vi "DB - Sort Item Names To DB.vi"(10 "DB Query Array":string[][](array[string]), 11 "ItemNames":string[][](array[string])) -> (2 "ItemNames":string[][](array[string]), 3 "DB Query Array":string[][](array[string]))   [LabVIEW 2020]
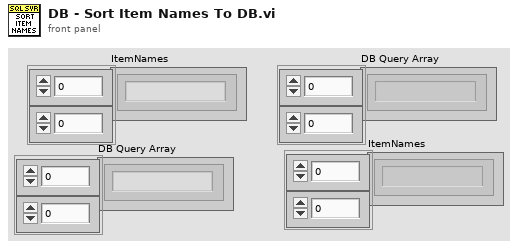
[diagram p1: front panel]
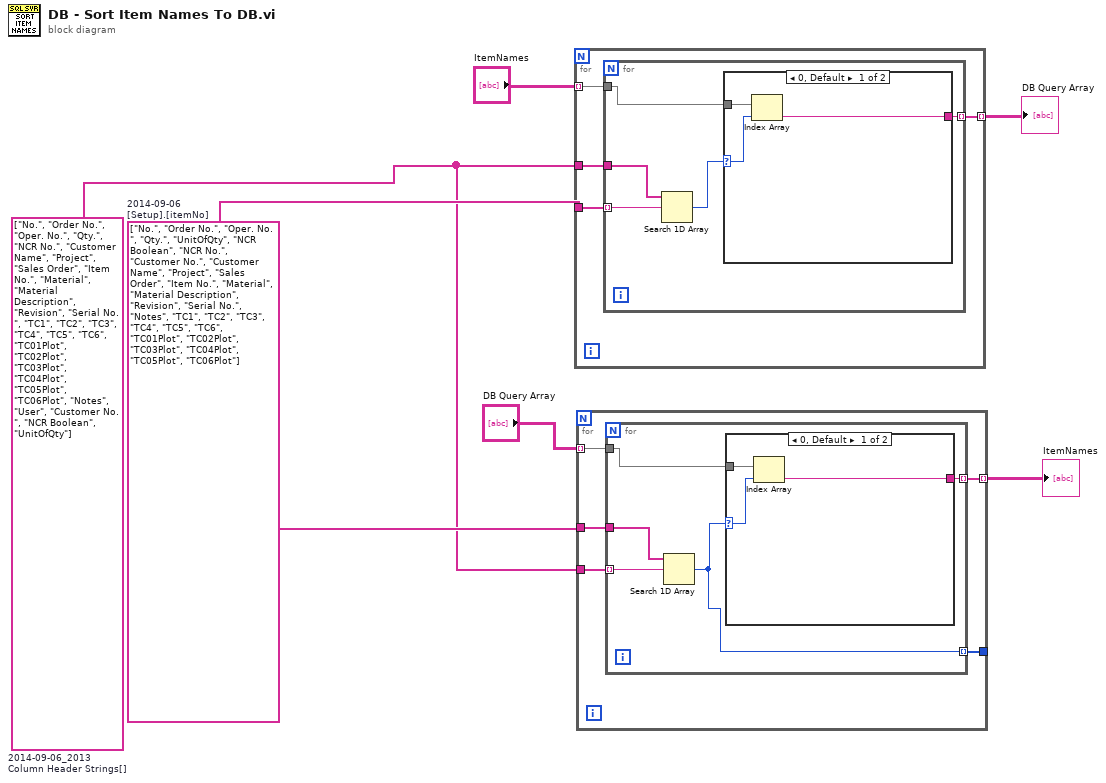
[diagram p0: block diagram]
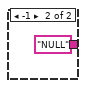
[diagram p2: hidden frame]
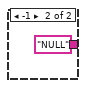
[diagram p3: hidden frame]
diagram:
  w2 = string[] ["No.", "Order No.", "Oper. No.", "Qty.", "NCR No.", "Customer Name", "Project", "Sales Order", "Item No.", "Material", "Material Description", "Revision", "Serial No.", "TC1", "TC2", "TC3", "TC4", "TC5", "TC6", "TC01Plot", "TC02Plot", "TC03Plot", "TC04Plot", "TC05Plot", "TC06Plot", "Notes", "User", "Customer No.", "NCR Boolean", "UnitOfQty"]  # 2014-09-06_2013 Column Header Strings[]
  w3 = string[] ["No.", "Order No.", "Oper. No.", "Qty.", "UnitOfQty", "NCR Boolean", "NCR No.", "Customer No.", "Customer Name", "Project", "Sales Order", "Item No.", "Material", "Material Description", "Revision", "Serial No.", "Notes", "TC1", "TC2", "TC3", "TC4", "TC5", "TC6", "TC01Plot", "TC02Plot", "TC03Plot", "TC04Plot", "TC05Plot", "TC06Plot"]  # 2014-09-06 [Setup].[itemNo]
  n1 = for {
    tunnel: "ItemNames" -> [w10] mode=indexing
    tunnel: w2 -> [w9]
    tunnel: w3 -> [w8]
    tunnel: [w7] -> w6 mode=indexing
    n2 = for {
      tunnel: w10 -> [w15]
      tunnel: w9 -> [w14]
      tunnel: w8 -> [w13] mode=indexing
      tunnel: [w12] -> w7 mode=indexing
      n3 = Search 1D Array(1D array=w14, element=w13) -> (index of element=w11:i32)  [unwired: 1 in]
      n4 = case shown="0, Default" w11 {
        selector: w11 -> [w17 _]
        tunnel: w15 -> [w18 _]
        tunnel: [w16 "NULL"] -> w12
        frame 0, Default {
          n5 = Index Array(array=w18, index=w17) -> (element=w16:string)
        }
        frame -1 {
        }
      }
    }
  }
  "DB Query Array" <- w6
  n6 = for {
    tunnel: "DB Query Array" -> [w24] mode=indexing
    tunnel: w3 -> [w23]
    tunnel: w2 -> [w22]
    tunnel: [w21] -> w1 mode=indexing
    tunnel: [w20] -> _
    n7 = for {
      tunnel: w24 -> [w29]
      tunnel: w23 -> [w28]
      tunnel: w22 -> [w27] mode=indexing
      tunnel: [w26] -> w21 mode=indexing
      tunnel: [w25] -> w20 mode=indexing
      n8 = Search 1D Array(1D array=w28, element=w27) -> (index of element=w25:i32)  [unwired: 1 in]
      n9 = case shown="0, Default" w25 {
        selector: w25 -> [w31 _]
        tunnel: w29 -> [w32 _]
        tunnel: [w30 "NULL"] -> w26
        frame 0, Default {
          n10 = Index Array(array=w32, index=w31) -> (element=w30:string)
        }
        frame -1 {
        }
      }
    }
  }
  "ItemNames" <- w1
